vi "MB Registers Manager Init.vi"(8 "error in (no error)":errorcluster) -> (0 "error out":errorcluster, 3 "Data Reference":T1)   [LabVIEW 2019, in "NI_modbus_upd.lvlib"]
uses:
  NI_modbus_upd.lvlib
  Ctl/Data Reference.ctl
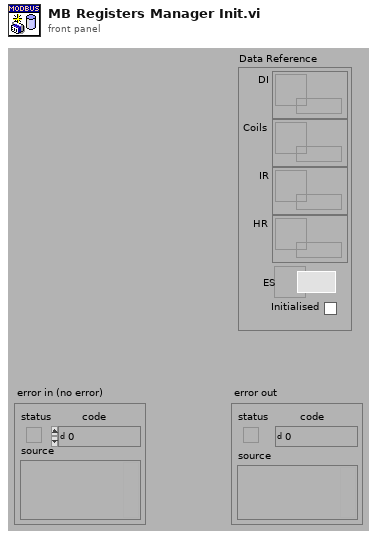
[diagram p1: front panel]
types:
  T1 = typedef "NI_modbus_upd.lvlib/Data Reference.ctl" = cluster{"DI":refnum<data-value>, "Coils":refnum<data-value>, "IR":refnum<data-value>, "HR":refnum<data-value>, "ES":refnum<data-value>, "Initialised":bool}
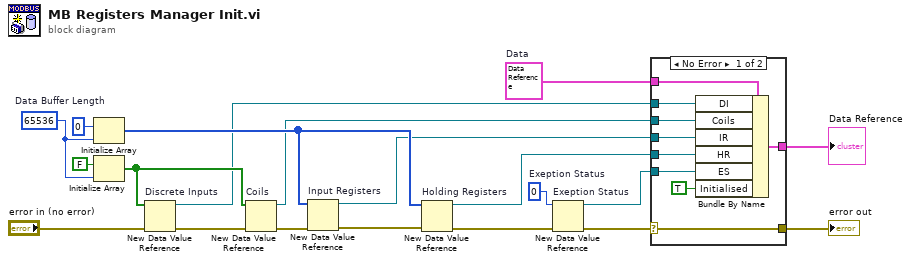
[diagram p0: block diagram]
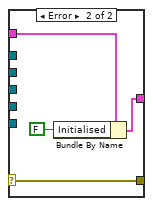
[diagram p2: hidden frame]
diagram:
  w2 = u8 0  # Exeption Status
  w11 = T1 {"DI"=refnum, "Coils"=refnum, "IR"=refnum, "HR"=refnum, "ES"=refnum, "Initialised"=FALSE}  # Data
  w6 = 65536  # Data Buffer Length
  n1 = Initialize Array(u16 0, w6) -> (w16:u16[])
  n2 = Initialize Array(FALSE, w6) -> (w14:bool[])
  n3 = New Data Value Reference "Discrete Inputs"(data value=w14, error in="error in (no error)") -> (data value reference=w10:refnum<data-value>, error out=w15:errorcluster)
  n4 = New Data Value Reference "Coils"(data value=w14, error in=w15) -> (data value reference=w9:refnum<data-value>, error out=w13:errorcluster)
  n5 = New Data Value Reference "Input Registers"(data value=w16, error in=w13) -> (data value reference=w8:refnum<data-value>, error out=w12:errorcluster)
  n6 = New Data Value Reference "Holding Registers"(data value=w16, error in=w12) -> (data value reference=w7:refnum<data-value>, error out=w5:errorcluster)
  n7 = New Data Value Reference "Exeption Status"(data value=w2, error in=w5) -> (data value reference=w3:refnum<data-value>, error out=w4:errorcluster)
  n8 = case shown="No Error" w4 {
    selector: w4 -> [w23 w33]
    tunnel: w11 -> [w29 w32]
    tunnel: w10 -> [w28 _]
    tunnel: w9 -> [w27 _]
    tunnel: w8 -> [w26 _]
    tunnel: w7 -> [w25 _]
    tunnel: [w24 w31] -> w1
    tunnel: [w23 w33] -> w19
    tunnel: w3 -> [w21 _]
    frame No Error {
      n9 = Bundle By Name(cluster=w29, "DI"=w28, "Coils"=w27, "IR"=w26, "HR"=w25, "ES"=w21, "Initialised"=TRUE) -> (w24:T1)
    }
    frame Error {
      n10 = Bundle By Name(cluster=w32, "Initialised"=FALSE) -> (w31:T1)
    }
  }
  "error out" <- w19
  "Data Reference" <- w1
